vi "Error Handler.vi"(8 "error in":errorcluster, 9 "Ignore Errors (Runtime)":i32[](array[numeric]), 10 "Exit on Error?":bool=TRUE) -> (0 "dup error in":errorcluster, 2 "Error?":bool)   [LabVIEW 2020, in "MHL.lvlib"]
doc: "Process an error that occurred in the state machine controlled by this library, either by ignoring it, or generating an \"Error\" message."
uses:
  MHL.lvlib
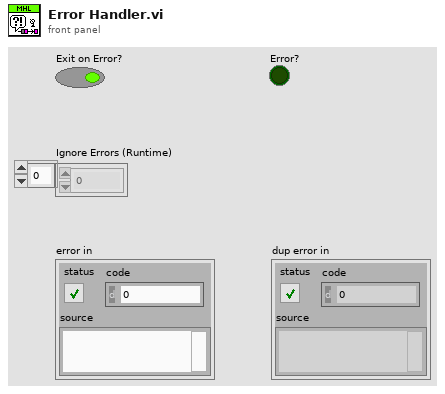
[diagram p1: front panel]
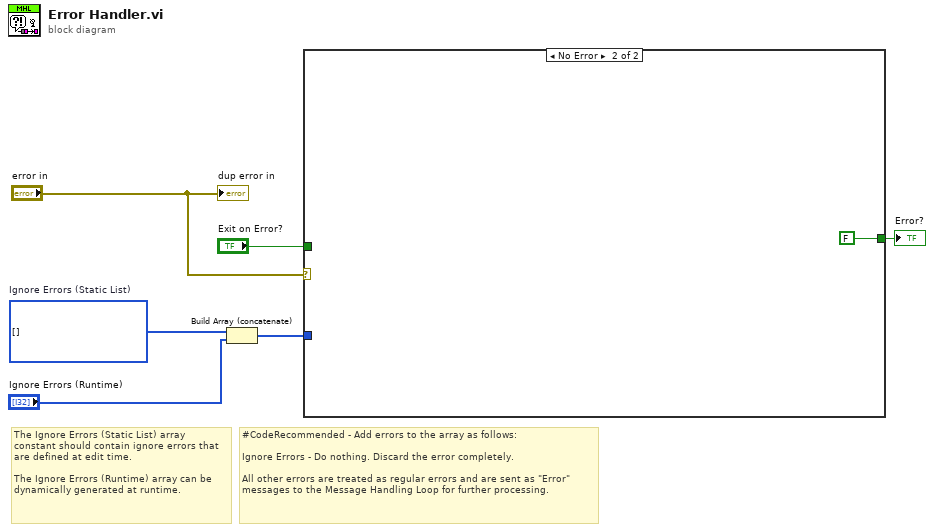
[diagram p0: block diagram]
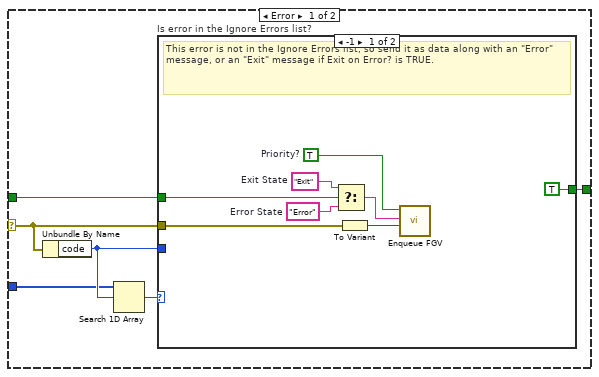
[diagram p2: hidden frame]
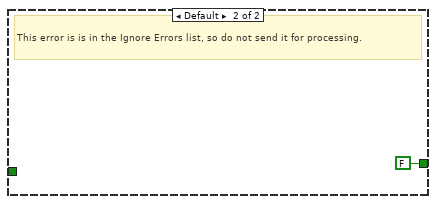
[diagram p3: hidden frame]
diagram:
  w1 = i32[] []  # Ignore Errors (Static List)
  # "The Ignore Errors (Static List) array constant should contain ignore errors that are defined at edit time.\n\nThe Ignore Errors (Runtime) array can be dynamically generated at runtime."
  # "#CodeRecommended - Add errors to the array as follows:\n\nIgnore Errors - Do nothing. Discard the error completely.\n\nAll other errors are treated as regular errors and are sent as \"Error\" messages to the Message Handling Loop for further processing."
  n1 = Build Array (concatenate)(w1, "Ignore Errors (Runtime)") -> (w6:i32[])
  n2 = case shown="No Error" "error in" {
    selector: "error in" -> [w10 _]
    tunnel: w6 -> [w9 _]
    tunnel: [w8 FALSE] -> w3
    tunnel: "Exit on Error?" -> [w7 _]
    frame Error {
      n3 = Unbundle By Name(w10) -> ("code"=w11:i32)
      n4 = Search 1D Array(1D array=w9, element=w11) -> (index of element=w12:i32)  [unwired: 1 in]
      n5 = case "Is error in the Ignore Errors list?" shown="-1" w12 {
        tunnel: w10 -> [w17 _]
        tunnel: w11 -> [_ _]
        tunnel: [TRUE FALSE] -> w8
        tunnel: w7 -> [w16 _]
        frame -1 {
          w15 = TRUE  # Priority?
          w18 = "Exit"  # Exit State
          w19 = "Error"  # Error State
          # "This error is not in the Ignore Errors list, so send it as data along with an \"Error\" message, or an \"Exit\" message if Exit on Error? is TRUE."
          n6 = Select(t=w18, s=w16, f=w19) -> (s? t:f=w14:string)
          n7 = To Variant(anything=w17) -> (Variant=w13:variant)
          n8 = call "Enqueue FGV.vi"("Message Data"=w13, "Message"=w14, "Priority?"=w15) -> ()  [unwired: 7 in, 2 out]
        }
        frame Default {
          # "This error is is in the Ignore Errors list, so do not send it for processing."
        }
      }
    }
    frame No Error {
    }
  }
  "Error?" <- w3
  "dup error in" <- "error in"
